vi "Change_Status_In_Case_Best_101-111-2.vi"(5 "error IN":errorcluster, 6 "[IN] Track group":T1, 7 "[IN] Indexes for Jumps":i32[](array[numeric]), 8 "[IN] Current Status":i16) -> (0 "error OUT":errorcluster, 3 "[OUT] Status of point after 101":i16)   [LabVIEW 2013]
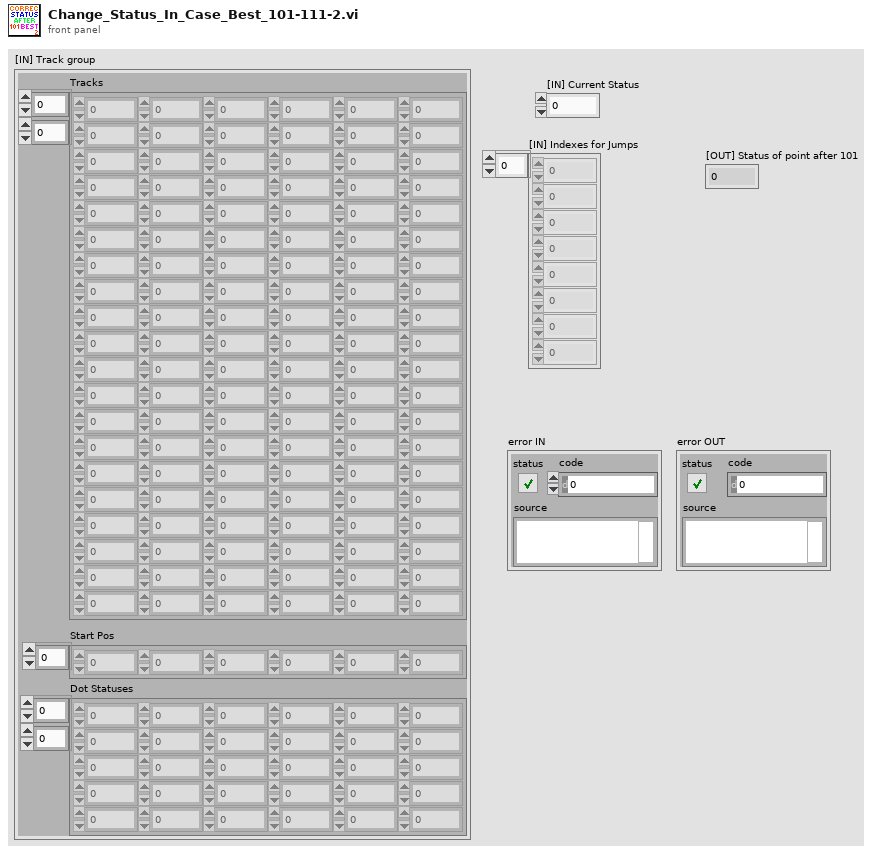
[diagram p1: front panel]
types:
  T1 = cluster{"Tracks":dbl[][], "Start Pos":i32[], "Dot Statuses":i16[][]}
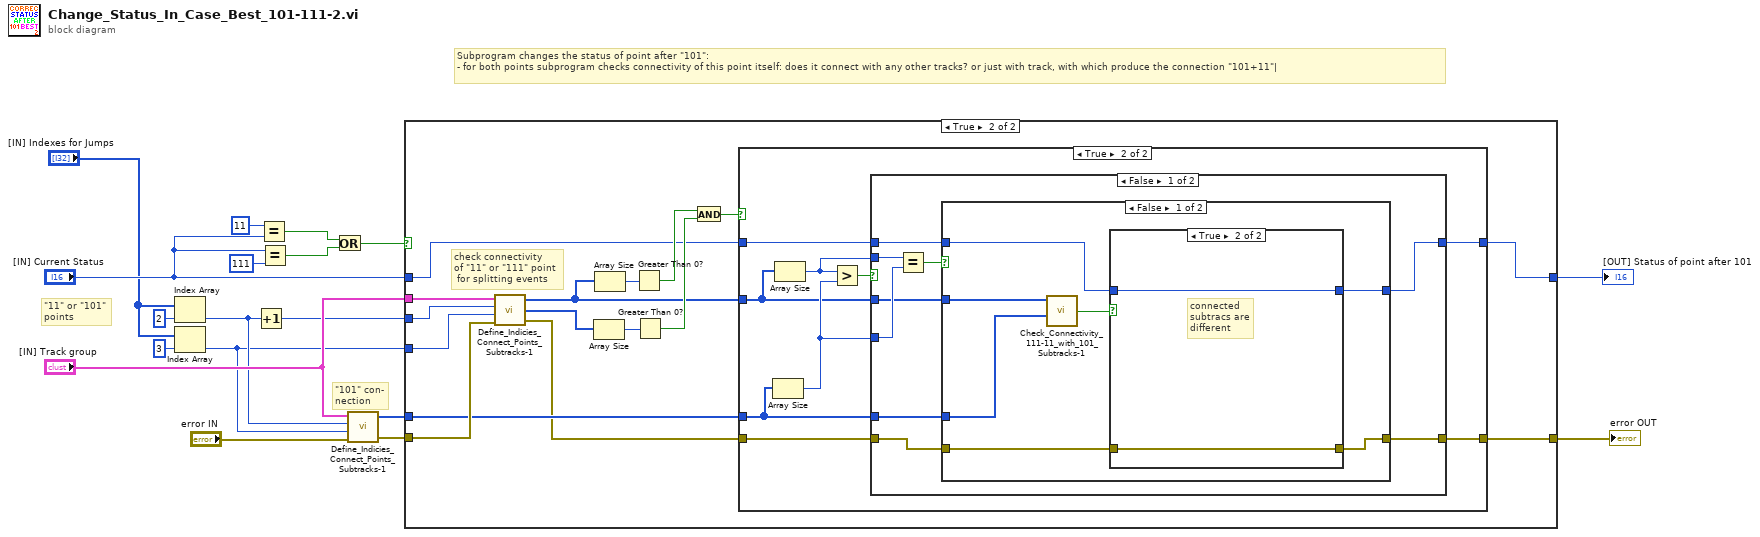
[diagram p0: block diagram]
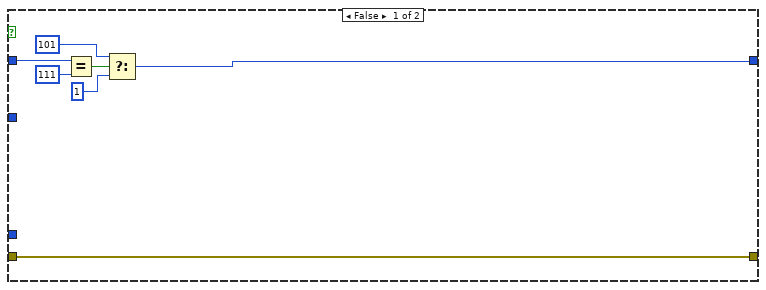
[diagram p3: hidden frame]
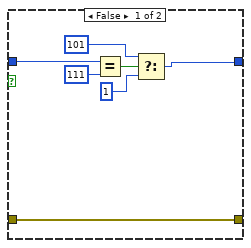
[diagram p4: hidden frame]
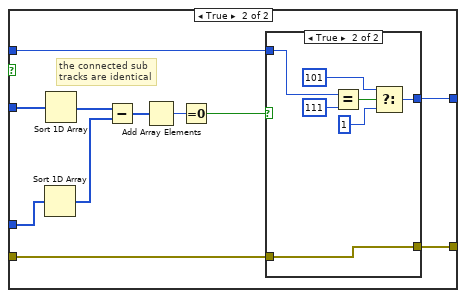
[diagram p5: hidden frame]
diagram:
  # "\"11\" or \"101\" \npoints"
  # "\"101\" con-\nnection"
  # "Subprogram changes the status of point after \"101\":\n- for both points subprogram checks connectivity of this point itself: does it connect with any other tracks? or just with track, with which produce the connection \"101+11\"|"
  n1 = Index Array(array="[IN] Indexes for Jumps", index=2) -> (element=w2:i32)
  n2 = Index Array(array="[IN] Indexes for Jumps", index=3) -> (element=w1:i32)
  n3 = Increment(x=w2) -> (x+1=w3:i32)
  n4 = Equal?(x=i16 11, y="[IN] Current Status") -> (x = y?=w10:bool)
  n5 = Equal?(x="[IN] Current Status", y=i16 111) -> (x = y?=w9:bool)
  n6 = Or(x=w10, y=w9) -> (x .or. y?=w8:bool)
  n7 = call "Define_Indicies_Connect_Points_Subtracks-1.vi"("error IN"="error IN", "[IN] Index of track with\n(problem displacement)"=w1, "[IN] Index of problem\ndisplacement inside track"=w2, "[IN] Track group"="[IN] Track group") -> ("error OUT"=w14:errorcluster, "[OUT] Index of connected\ntracks with problem dot"=w7:i32[])  [unwired: 1 out]
  n8 = case shown="True" w8 {
    tunnel: "[IN] Current Status" -> [w20 w28]
    tunnel: "[IN] Track group" -> [_ w36]
    tunnel: w14 -> [w19 w26]
    tunnel: [w20 w27] -> w16
    tunnel: [w19 w25] -> w17
    tunnel: w7 -> [_ w22]
    tunnel: w3 -> [_ w35]
    tunnel: w1 -> [_ w34]
    frame False {
    }
    frame True {
      # "check connectivity \nof \"11\" or \"111\" point\n for splitting events"
      n9 = call "Define_Indicies_Connect_Points_Subtracks-1.vi"("error IN"=w26, "[IN] Index of track with\n(problem displacement)"=w34, "[IN] Index of problem\ndisplacement inside track"=w35, "[IN] Track group"=w36) -> ("error OUT"=w21:errorcluster, "[OUT] Index of \nconnected dots\ninside the track"=w23:i32[], "[OUT] Index of connected\ntracks with problem dot"=w24:i32[])
      n10 = Array Size(array=w23) -> (size(s)=w32:i32)
      n11 = Array Size(array=w24) -> (size(s)=w33:i32)
      n12 = Greater Than 0?(x=w33) -> (x > 0?=w31:bool)
      n13 = Greater Than 0?(x=w32) -> (x > 0?=w30:bool)
      n14 = And(x=w31, y=w30) -> (x .and. y?=w29:bool)
      n15 = case shown="True" w29 {
        tunnel: w28 -> [w41 w51]
        tunnel: [w38 w50] -> w27
        tunnel: w21 -> [w37 w45]
        tunnel: [w37 w44] -> w25
        tunnel: w24 -> [_ w47]
        tunnel: w22 -> [_ w46]
        frame False {
          n16 = Equal?(x=w41, y=i16 111) -> (x = y?=w42:bool)
          n17 = Select(t=i16 101 ("y"), s=w42, f=i16 1) -> (s? t:f=w38:i16)
        }
        frame True {
          n18 = Array Size(array=w46) -> (size(s)=w48:i32)
          n19 = Array Size(array=w47) -> (size(s)=w49:i32)
          n20 = Greater?(x=w49, y=w48) -> (0:w52:bool)
          n21 = case shown="False" w52 {
            tunnel: [w55 w99] -> w50
            tunnel: w51 -> [w56 w99]
            tunnel: w49 -> [w61 _]
            tunnel: w48 -> [w60 _]
            tunnel: w47 -> [w58 _]
            tunnel: w46 -> [w57 _]
            tunnel: w45 -> [w54 w98]
            tunnel: [w53 w98] -> w44
            frame False {
              n22 = Equal?(x=w61, y=w60) -> (x = y?=w59:bool)
              n23 = case shown="False" w59 {
                tunnel: w58 -> [w68 w88]
                tunnel: w57 -> [w67 w87]
                tunnel: w56 -> [w65 w82]
                tunnel: [w64 w81] -> w55
                tunnel: w54 -> [w63 w80]
                tunnel: [w62 w79] -> w53
                frame False {
                  n24 = call "Check_Connectivity_111-11_with_101_Subtracks-1.vi"("[IN] Index of connected tracks \nwith \"101\" problem dot"=w67, "[IN] Index of connected tracks \nwith \"111\" or \"11\" problem dot"=w68) -> ("[OUT] Tracks aren't \nconnected after \"101\""=w66:bool)  [unwired: 4 in]
                  n25 = case shown="True" w66 {
                    tunnel: w65 -> [w71 w77]
                    tunnel: [w70 w77] -> w64
                    tunnel: w63 -> [w69 w76]
                    tunnel: [w69 w76] -> w62
                    frame False {
                      n26 = Equal?(x=w71, y=i16 111) -> (x = y?=w74:bool)
                      n27 = Select(t=i16 101 ("y"), s=w74, f=i16 1) -> (s? t:f=w70:i16)
                    }
                    frame True {
                      # "connected \nsubtracs are\ndifferent"
                    }
                  }
                }
                frame True {
                  # "the connected sub\ntracks are identical"
                  n28 = Sort 1D Array(array=w87) -> (sorted array=w85:i32[])
                  n29 = Sort 1D Array(array=w88) -> (sorted array=w86:i32[])
                  n30 = Subtract(x=w86, y=w85) -> (x-y=w84:i32[])
                  n31 = Add Array Elements(numeric array=w84) -> (sum=w83:i32)
                  n32 = Equal To 0?(x=w83) -> (x = 0?=w78:bool)
                  n33 = case shown="True" w78 {
                    tunnel: w82 -> [w90 w93]
                    tunnel: [w90 w92] -> w81
                    tunnel: w80 -> [w89 w91]
                    tunnel: [w89 w91] -> w79
                    frame False {
                      # "connected \nsubtracs are\ndifferent"
                    }
                    frame True {
                      n34 = Equal?(x=w93, y=i16 111) -> (x = y?=w96:bool)
                      n35 = Select(t=i16 101 ("y"), s=w96, f=i16 1) -> (s? t:f=w92:i16)
                    }
                  }
                }
              }
            }
            frame True {
            }
          }
        }
      }
    }
  }
  "error OUT" <- w17
  "[OUT] Status of point after 101" <- w16
